vi "Set Mode.vi"(8 "error in (no error)":errorcluster, 10 "Mode":T1 items=["Operator"=0, "Engineering"=1, "Verification"=6], 11 "App Properties in":refnum<class "App Properties.lvclass">) -> (0 "error out":errorcluster, 3 "App Properties out":refnum<class "App Properties.lvclass">)   [LabVIEW 2015, in "Application.lvlib" / "App Properties.lvclass"]
uses:
  App Properties.lvclass
  Class/typedefs/Op Mode -- Enum.ctl
  App Properties.lvclass/App Properties.ctl
  Class/Application.lvclass
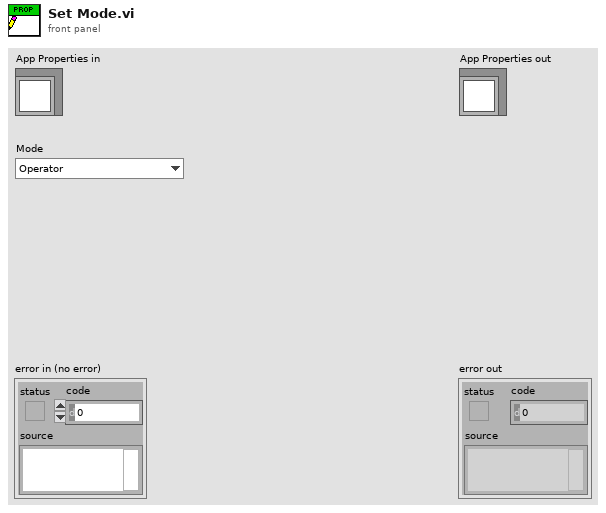
[diagram p1: front panel]
types:
  T1 = typedef "Application.lvlib/Application.lvclass/Op Mode -- Enum.ctl" = u16
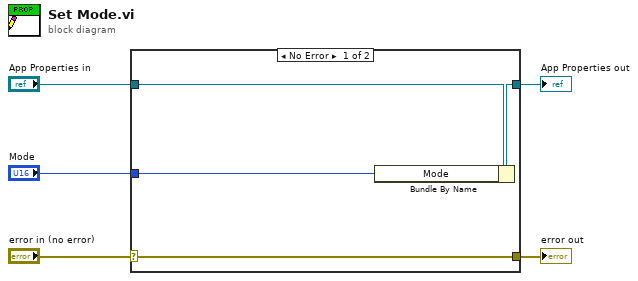
[diagram p0: block diagram]
diagram:
  n1 = case shown="No Error" "error in (no error)" {
    selector: "error in (no error)" -> [w9 w10]
    tunnel: [w9 w10] -> w4
    tunnel: [w7 w11] -> w2
    tunnel: "App Properties in" -> [w8 w11]
    tunnel: "Mode" -> [w6 _]
    frame No Error {
      n2 = Bundle By Name(cluster=w8, "Mode"=w6) -> (w7:refnum<class "App Properties.lvclass">)
    }
    frame Error {
    }
  }
  "error out" <- w4
  "App Properties out" <- w2
